vi "TDC_calcHbtModelFct.vi"(8 "Error In":errorcluster, 9 "fct in":u64, 10 "Parameters":dbl[](array[numeric]), 11 "Function Type":u16(ring) items=["None", "Coherent", "Thermal", "Single", "Antibunch", "Thermal+Jitter", "Single+Jitter", "Antibunch+Jitter", "Thermal+Offset", "Single+Offset", "Antibunch+Offset", "Thermal+Jitter+Offs", "Single+Jitter+Offs", "Antibunch+Jitter+Offs"]) -> (0 "Error Out":errorcluster, 1 "fct out":i32)   [LabVIEW 2011]
uses:
  tdcbase.dll
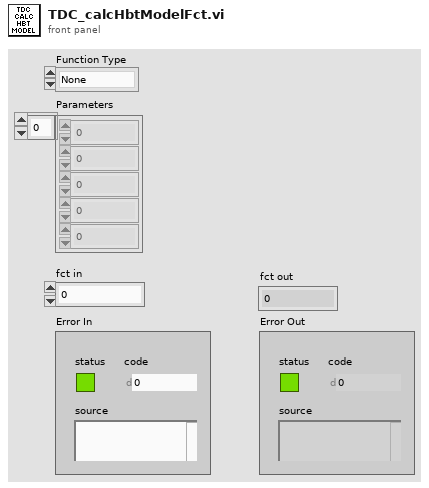
[diagram p1: front panel]
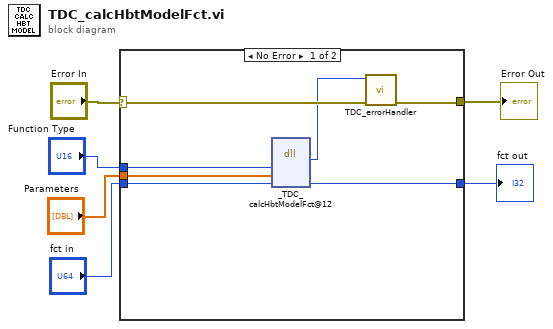
[diagram p0: block diagram]
diagram:
  n1 = case shown="No Error" "Error In" {
    selector: "Error In" -> [w12 w15]
    tunnel: [w11 w15] -> w5
    tunnel: [w13 w14] -> w4
    tunnel: "Function Type" -> [w9 _]
    tunnel: "Parameters" -> [w8 _]
    tunnel: "fct in" -> [w7 w14]
    frame No Error {
      n2 = dll-call lib="X:/tdcbase.dll" fn="_TDC_calcHbtModelFct@12"("fctType"=w9, "params"=w8, "fct"=w7) -> ("return type"=w10:i32, "fct"=w13:u64)  [unwired: 5 in, 2 out]
      n3 = call "TDC_errorHandler.vi"("Error In"=w12, "TDC Return Code"=w10) -> ("Error Out"=w11:errorcluster)  [unwired: 9 in]
    }
    frame Error {
    }
  }
  "Error Out" <- w5
  "fct out" <- w4
